vi "WriteStoreData (2).vi"(1 "Spots":T1[](array[typedef]) {"F2-Value overall" format="%.2f"; "tauerror" format="%.2f"; "Lifetime[ns]" format="%.2f"; "F2-Value TAC" format="%.2f"}, 2 "Enum":enum16{"Save", "Control"}(ring), 3 "Image Path":refnum<vi>) -> (0 "already x spots":i16)   [LabVIEW 2009]
uses:
  spotproperties.ctl
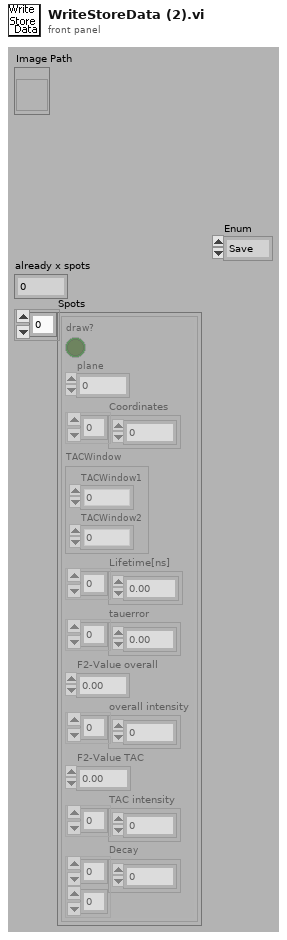
[diagram p1: front panel]
types:
  T1 = typedef "spotproperties.ctl" = cluster{"draw?":bool, "plane":u32, "Coordinates":i32[], "TACWindow":cluster{"TACWindow1":i32, "TACWindow2":i32}, "Lifetime[ns]":ext[], "tauerror":dbl[], "F2-Value overall":dbl, "overall intensity":u32[], "F2-Value TAC":dbl, "TAC intensity":u32[], "Decay":u32[][]}
  T2 = enum16{"Display", "change", "Get", "Set", "Set Ken"}
  T3 = enum16{"open", "open or create", "create or replace", "create", "open (read only)"}
  T4 = enum16{"read/write", "read-only", "write-only", "write-only (truncate)"}
  T5 = typedef "Settings.ctl" = cluster{"threshold":cluster{"max":u32, "min":u32}, "RGB or false color":bool, "16bit":bool, "log/lin axis":u16, "spotsize button":bool, "Pixelsize":u16, "autoscale x":bool, "autoscale y":bool, "correlation":bool, "ADC-Resolution":i32, "F2-lifetime":cluster{"display tau":bool, "display F2":bool, "Palette Number lifetime":enum32{"Gray", "Binary", "Gradient", "Rainbow", "Temperature"}, "Palette Number F2":enum32{"Gray", "Binary", "Gradient", "Rainbow", "Temperature"}, "max tau-Value":dbl, "min tau-Value":dbl, "max F2-Value":dbl, "min F2-Value":dbl}, "TAC-Window 1":u16, "TAC-Window 2":u16, "false color palette":cluster{"1":u32, "2":u32, "3":u32, "4":u32, "5":u32, "6":u32, "7":u32, "8":u32, "8 2":u32, "8 3":u32, "8 4":u32, "8 5":u32}, "rebinning":dbl}
  T6 = typedef "FIFOSettings_BH.ctt" = cluster{"Measurement":cluster{"Binning (ms)":sgl, "External Trigger Condition":u16, "Stop Condition:":u16, "Stop Count":dbl, "Buffer Size (Photons)":u16, "No of Channels":u16, "Ext Latch Delay":i16}, "ADC":cluster{"Module":u16, "ADC Resolution":i32, "Dither Range":i16, "Count Increment":i16, "Macro Time Clock":i16}, "SYNC":cluster{"SYNC ZC Level (mV)":sgl, "SYNC Freq Divider":i16, "SYNC Holdoff (ns)":sgl, "SYNC Threshold (mV)":sgl}, "TAC":cluster{"TAC Range (ns)":sgl, "TAC Gain":i16, "TAC Offset (%)":sgl, "TAC Limit Low (%)":sgl, "TAC Limit High (%)":sgl}, "CFD":cluster{"CFD Limit Low (mV)":sgl, "CFD Limit High (mV)":sgl, "CFD ZC Level (mV)":sgl, "CFD Holdoff (ns)":sgl}}
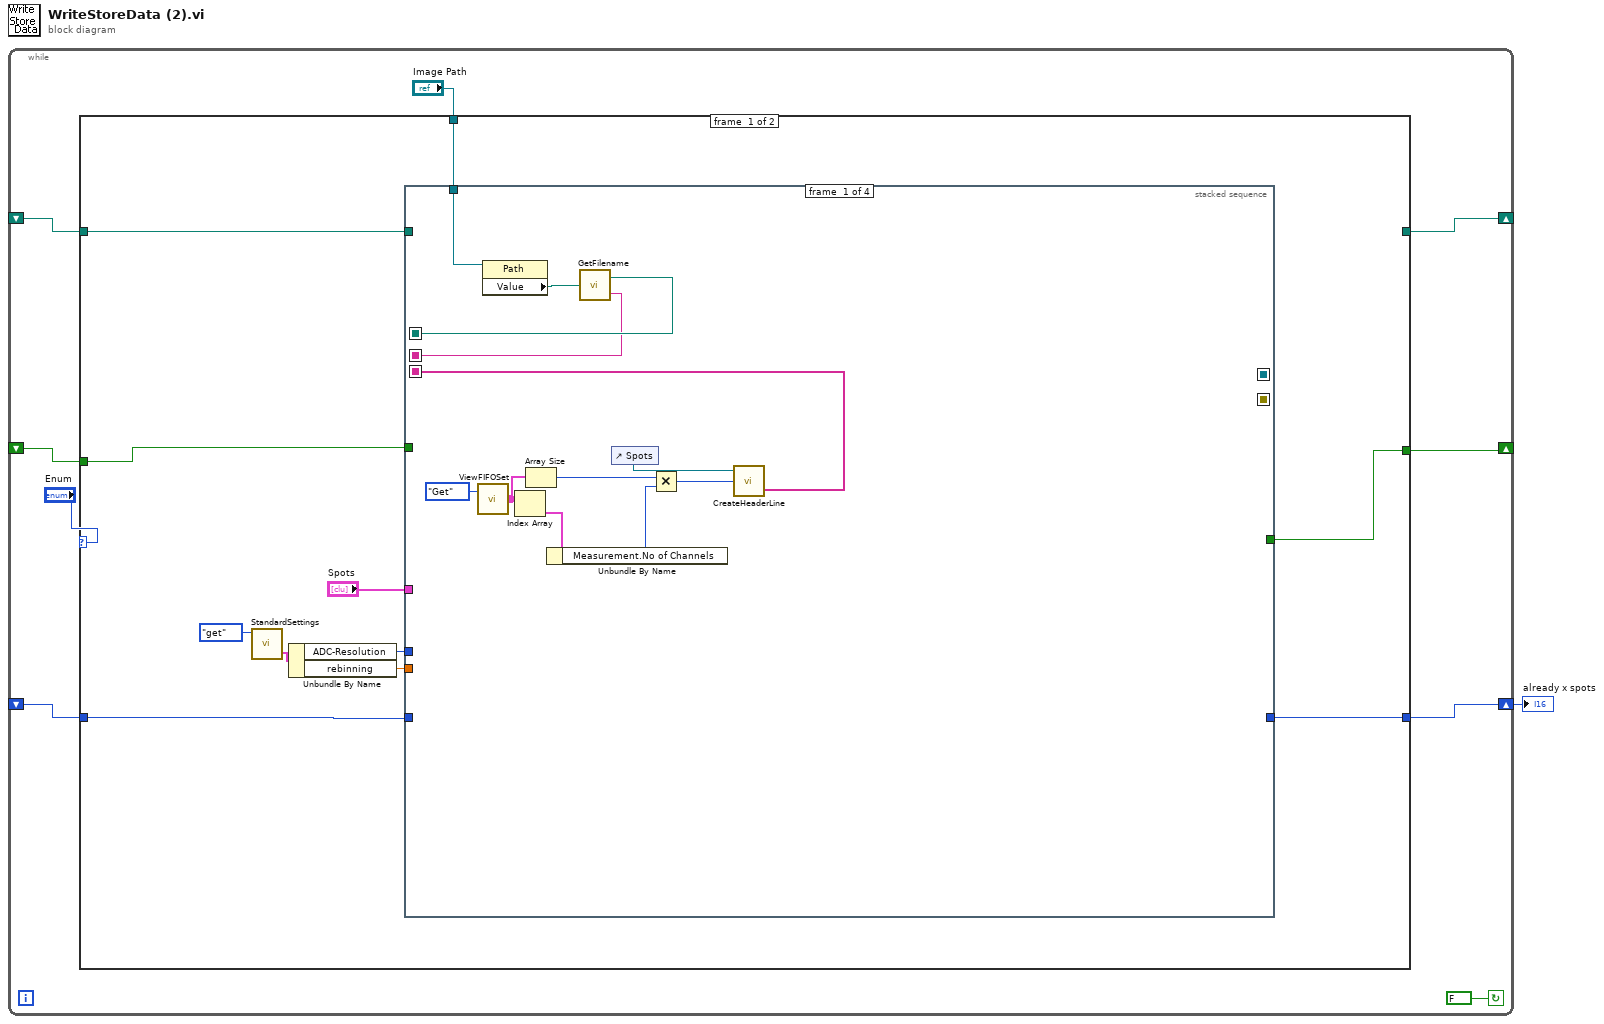
[diagram p0: block diagram]
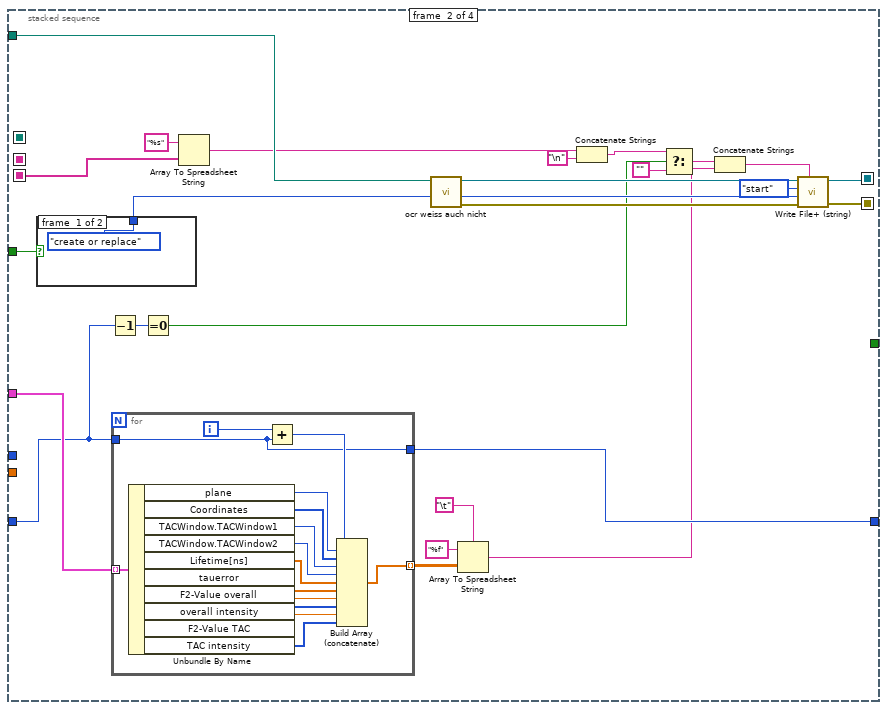
[diagram p2: hidden frame]
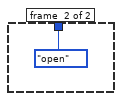
[diagram p3: hidden frame]
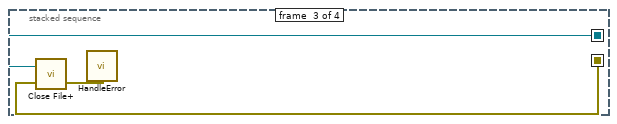
[diagram p4: hidden frame]
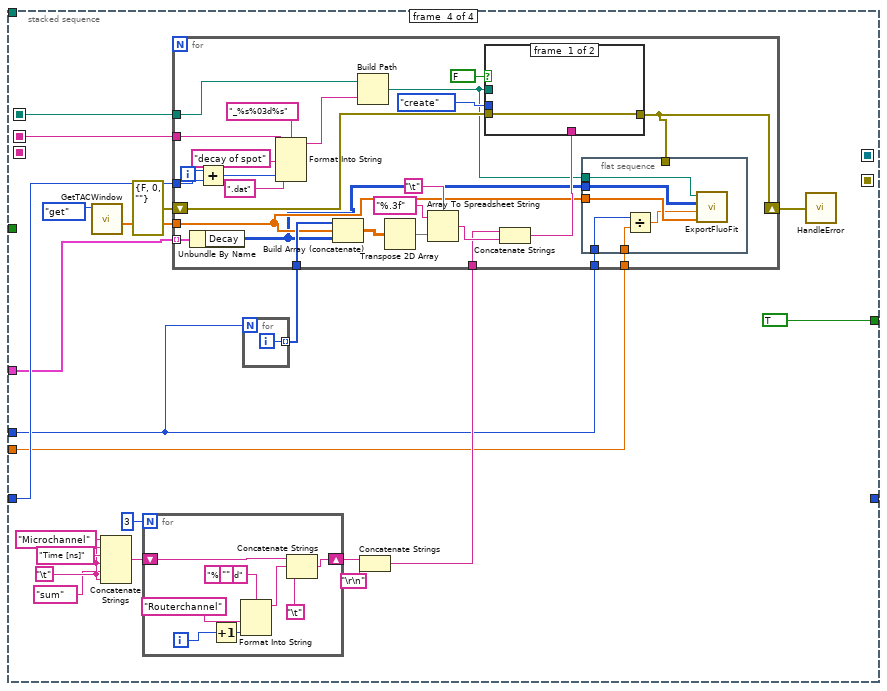
[diagram p5: hidden frame]
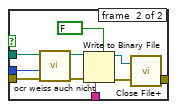
[diagram p6: hidden frame]
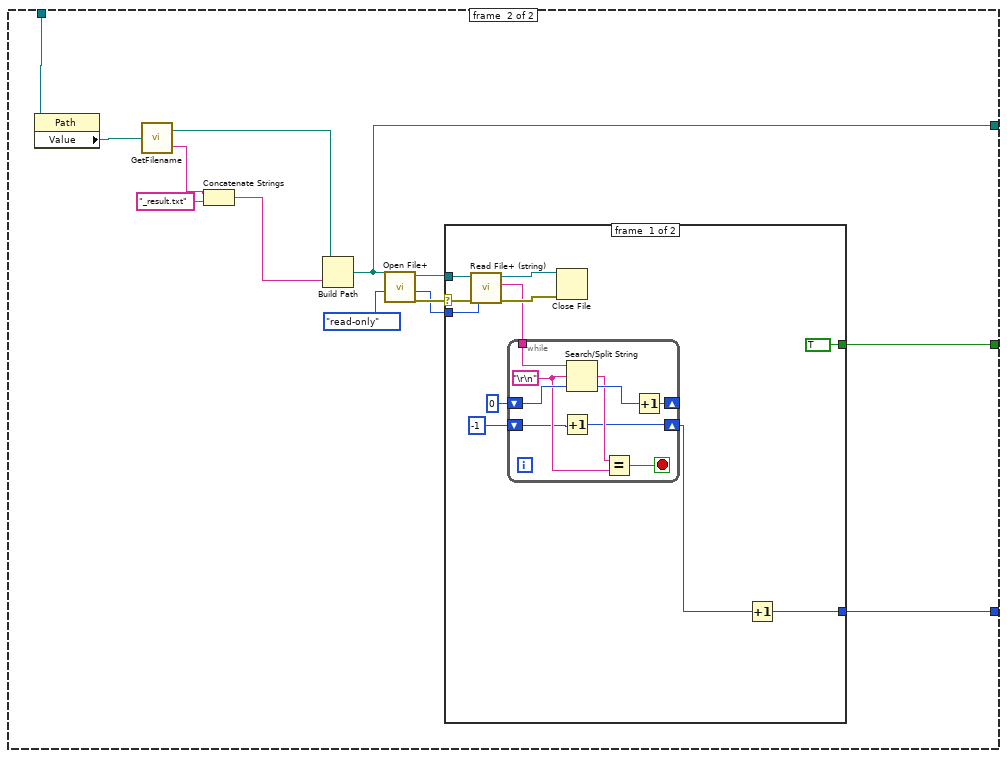
[diagram p7: hidden frame]
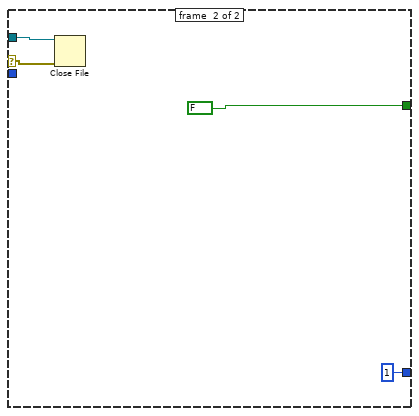
[diagram p8: hidden frame]
diagram:
  n1 = while {
    shift-right: [w8] -> _
    shift-left: _ -> [w7]
    shift-right: [w6] -> w1
    shift-left: _ -> [w5]
    shift-right: [w4] -> _
    shift-left: _ -> [w3]
    stop <- FALSE continue-if-true
    n2 = case shown="\"Save\", Default" "Enum" {
      tunnel: [w21 w166] -> w8
      tunnel: w7 -> [w20 _]
      tunnel: [w19 w154] -> w6
      tunnel: w5 -> [w12 _]
      tunnel: [_ w156] -> w4
      tunnel: w3 -> [w18 _]
      tunnel: "Image Path" -> [w17 w155]
      frame #0 {
        n3 = call "StandardSettings.vi"("Enum"=enum16{"Load", "get", "Save", "set"}."get") -> ("StandardSettings"=w15:T5)  [unwired: 4 in]
        n4 = Unbundle By Name(w15) -> ("ADC-Resolution"=w14:i32, "rebinning"=w11:dbl)
        n5 = stacked-sequence {
          seq-local: [w33 _ _ _] -> [_ _ _ w100]
          seq-local: [w30 _ _ _] -> [_ _ _ w88]
          seq-local: [w28 _ _ _] -> [_ w45 _ _]
          seq-local: [_ w58 _ _] -> [_ _ w79 _]
          seq-local: [_ w57 _ _] -> [_ _ w78 _]
          tunnel: "Spots" -> [_ w56 _ w85]
          tunnel: [_ _ _ TRUE] -> w21
          tunnel: w20 -> [_ w49 _ _]
          tunnel: [_ w48 _ _] -> w19
          tunnel: w12 -> [_ w41 _ w92]
          tunnel: w18 -> [_ w46 _ _]
          tunnel: w17 -> [w32 _ _ _]
          tunnel: w14 -> [_ _ _ w80]
          tunnel: w11 -> [_ _ _ w81]
          frame #0 {
            n6 = call "ViewFIFOSet.vi"("Enum"=T2."Get") -> ("FIFO Settings (Array)"=w23:T6[])  [unwired: 1 in]
            n7 = property class="Path"(reference=w32) -> ("Value"=w31:path)  [unwired: 1 in, 2 out]
            n8 = Index Array(array=w23) -> (element=w26:T6)  [unwired: 1 in]
            n9 = Array Size(array=w23) -> (size(s)=w24:i32)
            n10 = Unbundle By Name(w26) -> ("Measurement.No of Channels"=w25:u16)
            n11 = call "GetFilename.vi"("Value"=w31) -> ("base path"=w33:path, "name"=w30:string)
            n12 = control-ref of="Spots"() -> (w29:refnum<vi>)
            n13 = Multiply(x=w24, y=w25) -> (x*y=w22:i32)
            n14 = call "CreateHeaderLine.vi"("No of channels"=w22, "Spots 3"=w29) -> ("Headline array"=w28:string[])  [unwired: 2 in]
          }
          frame #1 {
            n15 = case shown="True" w49 {
              tunnel: [T3."create or replace" ("function (open:0)") T3."open" ("function (open:0)")] -> w59
              frame #0 {
              }
              frame #1 {
              }
            }
            n16 = Decrement(x=w41) -> (x-1=w42:i16)
            n17 = for {
              tunnel: w56 -> [w76] mode=indexing
              tunnel: [w75] -> w55 mode=indexing
              tunnel: [w72] -> w48
              tunnel: w41 -> [w72]
              i -> [w74]
              n18 = Unbundle By Name(w76) -> ("plane"=w71:u32, "Coordinates"=w70:i32[], "TACWindow.TACWindow1"=w69:i32, "TACWindow.TACWindow2"=w68:i32, "Lifetime[ns]"=w67:ext[], "tauerror"=w66:dbl[], "F2-Value overall"=w65:dbl, "overall intensity"=w64:u32[], "F2-Value TAC"=w63:dbl, "TAC intensity"=w62:u32[])
              n19 = Add(x=w74, y=w72) -> (x+y=w73:i32)
              n20 = Build Array (concatenate)(w73, w71, w70, w69, w68, w67, w66, w65, w64, w63, w62) -> (w75:ext[])
            }
            n21 = Equal To 0?(x=w42) -> (x = 0?=w40:bool)
            n22 = Array To Spreadsheet String(array=w45, 3:"%s" ("format string")) -> (spreadsheet string=w43:string)  [unwired: 1 in]
            n23 = call "ocr weiss auch nicht.vi"("function (open:0)"=w59, "file path"=w46) -> ("error out"=w52:errorcluster, "file size (bytes)"=w50:i32, "refnum"=w53:refnum<file>)  [unwired: 6 in, 1 out]
            n24 = Array To Spreadsheet String(delimiter (Tab)="\t", array=w55, 3:"%f" ("format string")) -> (spreadsheet string=w36:string)
            n25 = Concatenate Strings(w43, "\n") -> (w39:string)
            n26 = Select(t=w39, s=w40, f="") -> (s? t:f=w37:string)
            n27 = Concatenate Strings(w37, w36) -> (w35:string)
            n28 = call "Write File+ (string).vi"("string"=w35, "error in (no error)"=w52, "pos offset (bytes:0)"=w50, "pos mode (rel. to end:1)"=enum16{"start", "end", "current"}."start", "refnum"=w53) -> ("error out"=w57:errorcluster, "dup refnum"=w58:refnum<file>)  [unwired: 2 in, 1 out]
          }
          frame #2 {
            n29 = call "Close File+.vi"("error in (no error)"=w78, "refnum"=w79) -> ("error out"=w77:errorcluster)  [unwired: 3 in, 2 out]
            n30 = call "HandleError.vi"("error in (no error)"=w77) -> ()
          }
          frame #3 {
            w87 = "\t"
            n31 = call "GetTACWindow.vi"("Enum"=enum16{"ini", "get", "quick"}."get") -> ("x-values"=w82:dbl[])  [unwired: 1 in, 8 out]
            n32 = Concatenate Strings("Microchannel" ("string"), w87, "Time [ns]" ("string"), w87, "sum" ("string"), w87) -> (w94:string)
            n33 = for {
              N: 3 -> [_]
              shift-right: [w109] -> w98
              shift-left: w94 -> [w108]
              i -> [w106]
              (unwired) "%s %d" ("format string")
              n34 = Increment(x=w106) -> (x+1=w105:i32)
              n35 = Format Into String(format string="", "Routerchannel", w105) -> (resulting string=w103:string)  [unwired: 2 in, 1 out]
              n36 = Concatenate Strings(w108, w103, "\t") -> (w109:string)
            }
            n37 = for {
              N: w80 -> [_]
              tunnel: [w101] -> w90 mode=indexing
              i -> [w101]
            }
            n38 = Concatenate Strings(w98, "\r\n") -> (w97:string)
            n39 = for {
              tunnel: w85 -> [w136] mode=indexing
              tunnel: w100 -> [w135]
              tunnel: w82 -> [w116]
              shift-right: [w114] -> w83
              shift-left: errorcluster {"status"=FALSE, "code"=0, "source"=""} ("error out") -> [w130]
              tunnel: w97 -> [w127]
              tunnel: w92 -> [w122]
              tunnel: w88 -> [w117]
              tunnel: w90 -> [w118]
              tunnel: w81 -> [w111]
              tunnel: w80 -> [w110]
              i -> [w123]
              n40 = Unbundle By Name(w136) -> ("Decay"=w112:u32[][])
              n41 = Add(x=w123, y=w122) -> (x+y=w121:i32)
              n42 = Format Into String(format string="_%s%03d%s", initial string=w117, "decay of spot", w121, ".dat" ("replace string (\"\")")) -> (resulting string=w125:string)  [unwired: 1 in, 1 out]
              n43 = Build Array (concatenate)(w118, w116, w112) -> (w133:dbl[][])
              n44 = Build Path(base path=w135, name or relative path=w125) -> (appended path=w115:path)
              n45 = Transpose 2D Array(2D array=w133) -> (transposed array=w132:dbl[][])
              n46 = Array To Spreadsheet String(delimiter (Tab)="\t", array=w132, 3:"%.3f" ("format string")) -> (spreadsheet string=w129:string)
              n47 = Concatenate Strings(w127, w129) -> (w128:string)
              n48 = case shown="True" FALSE {
                tunnel: w130 -> [w137 w143]
                tunnel: w128 -> [_ w142]
                tunnel: T3."create" ("function (open:0)") -> [_ w141]
                tunnel: w115 -> [_ w140]
                tunnel: [w137 w139] -> w114
                frame #0 {
                }
                frame #1 {
                  n49 = call "ocr weiss auch nicht.vi"("error in (no error)"=w143, "function (open:0)"=w141, "file path"=w140) -> ("error out"=w144:errorcluster, "refnum"=w145:refnum<file>)  [unwired: 5 in, 2 out]
                  n50 = Write to Binary File(file (use dialog)=w145, data=w142, error in=w144, 5:FALSE ("prepend array or string size? (T)")) -> (refnum out=w146:refnum<file>, error out=w147:errorcluster)  [unwired: 2 in, 1 out]
                  n51 = call "Close File+.vi"("error in (no error)"=w147, "refnum"=w146) -> ("error out"=w139:errorcluster)  [unwired: 3 in, 2 out]
                }
              }
              n52 = flat-sequence {
                tunnel: w116 -> [w153]
                tunnel: w115 -> [w152]
                tunnel: w114 -> [_]
                tunnel: w112 -> [w151]
                tunnel: w111 -> [w150]
                tunnel: w110 -> [w149]
                frame #0 {
                  n53 = Divide(x=w149, y=w150) -> (x/y=w148:dbl)
                  n54 = call "ExportFluoFit.vi"("time in"=w153, "# of lines"=w148, "lifetimes"=w151, "Lifetime Export Path (ASCII-File)"=w152) -> ()  [unwired: 1 in]
                }
              }
            }
            n55 = call "HandleError.vi"("error in (no error)"=w83) -> ()
          }
        }
      }
      frame #1 {
        n56 = property class="Path"(reference=w155) -> ("Value"=w161:path)  [unwired: 1 in, 2 out]
        n57 = call "GetFilename.vi"("Value"=w161) -> ("base path"=w159:path, "name"=w160:string)
        n58 = Concatenate Strings(w160, "_result.txt" ("string")) -> (w157:string)
        n59 = Build Path(base path=w159, name or relative path=w157) -> (appended path=w156:path)
        n60 = call "Open File+.vi"("open mode (read-only:1)"=T4."read-only", "file path (\" \")"=w156) -> ("error out"=w163:errorcluster, "file size (bytes)"=w162:i32, "refnum"=w164:refnum<file>)  [unwired: 6 in, 1 out]
        n61 = case shown="No Error" w163 {
          selector: w163 -> [w175 w187]
          tunnel: w164 -> [w176 w188]
          tunnel: [TRUE FALSE] -> w166
          tunnel: [w167 i16 1] -> w154
          tunnel: w162 -> [w169 _]
          frame #0 {
            n62 = call "Read File+ (string).vi"("count"=w169, "error in (no error)"=w175, "refnum"=w176) -> ("error out"=w173:errorcluster, "string"=w172:string, "dup refnum"=w174:refnum<file>)  [unwired: 4 in, 2 out]
            n63 = while {
              shift-right: [w178] -> _
              shift-left: 0 ("offset of match") -> [w184]
              shift-right: [w179] -> w168
              shift-left: i16 -1 -> [w180]
              tunnel: w172 -> [w186]
              stop <- w181 stop-if-true
              w182 = "\r\n"
              n64 = Increment(x=w180) -> (x+1=w179:i16)
              n65 = Search/Split String(string=w186, search string/char (-)=w182, offset (0)=w184) -> (match + rest of string=w183:string, offset of match=w185:i32)  [unwired: 1 out]
              n66 = Equal?(x=w183, y=w182) -> (x = y?=w181:bool)
              n67 = Increment(x=w185) -> (x+1=w178:i32)
            }
            n68 = Close File(refnum=w174, error in=w173) -> ()  [unwired: 2 out]
            n69 = Increment(x=w168) -> (x+1=w167:i16)
          }
          frame #1 {
            n70 = Close File(refnum=w188, error in=w187) -> ()  [unwired: 2 out]
          }
        }
      }
    }
  }
  "already x spots" <- w1
